vi "Set Pressure Units.vi"(8 "error in (no error)":errorcluster, 10 "Pressure Units (28: Pound-force pre square inch)":u32(ring)=28 items=["Unitless", "Frequency in units of hertz", "Frequency in units of kilohertz", "Frequency in units of megahertz", "Volts in units of microvolts", "Volts in units of millivolts", "Volts in units of volts", "Volts in units of kilovolts", "Current in units of microamperes", "Current in units of milliamps", "Current in units of amps", "Percent", "Parts-per-million", "Volts in units of decibels referenced to 1 milliwatt into 600 W load", "Resistance in units of ohms", "Resistance in units of kilohms", "Resistance in units of megohms", "Capacitance in units of nanofarads", "Capacitance in units of picofarads", "Capacitance in units of  microfarads", "Capacitance in units of millifarads", "Capacitance in units of farads", "Temperature in degrees Celsius", "Temperature in degrees Fahrenheit", "Period in units of nanoseconds", "Period in units of microseconds", "Period in units of milliseconds", "Period in units of seconds", "Pound-force pre square inch", "Meters of mercury", "Inches of mercury", "Inches of water", "Feet of water", "Meters of water", "Bar", "Pascal", "Grams per centimeter squared", "Inches of water @ 60 degrees Farhenheit", "Decibels"], 11 "VISA resource name":refnum<visa-resource-name>) -> (0 "error out":errorcluster, 3 "VISA resource name out":refnum<visa-resource-name>)   [LabVIEW 2011, in "Fluke 5XXX Series Multicalibrators.lvlib"]
doc: "This VI sets the pressure display units.\n\nNote:\n\nThis VI is available only for instrument model 5520A with option 700P (pressure modules)."
uses:
  Fluke 5XXX Series Multicalibrators.lvlib
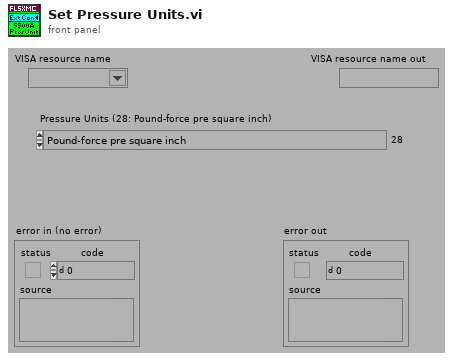
[diagram p1: front panel]
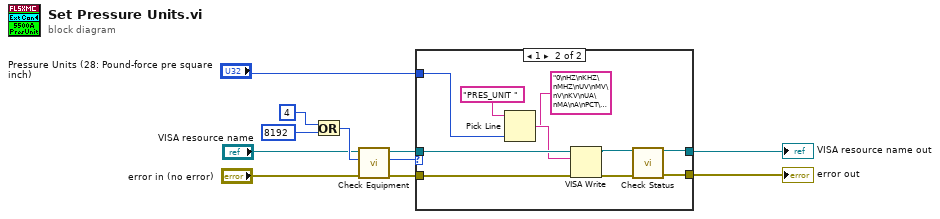
[diagram p0: block diagram]
diagram:
  n1 = Or(x=4 ("Numeric"), y=8192 ("Numeric")) -> (x .or. y?=w11:i32)
  n2 = call "Check Equipment.vi"("error in (no error)"="error in (no error)", "Bit Mask"=w11, "VISA resource name"="VISA resource name") -> ("error out"=w10:errorcluster, "Present?"=w9:u32, "VISA resource name out"=w8:refnum<visa-resource-name>)  [unwired: 6 in]
  n3 = case shown="1" w9 {
    tunnel: "Pressure Units (28: Pound-force pre square inch)" -> [_ w19]
    tunnel: [w12 w15] -> w4
    tunnel: w10 -> [w13 w22]
    tunnel: w8 -> [w12 w21]
    tunnel: [w13 w18] -> w5
    frame 0, Default {
    }
    frame 1 {
      n4 = Pick Line(string ("")="PRES_UNIT " ("Reset Command"), multi-line string="0\nHZ\nKHZ\nMHZ\nUV\nMV\nV\nKV\nUA\nMA\nA\nPCT\nPPM\nDBM\nOHM\nKOHM\nMOHM\nNF\nPF\nUF\nMF\nF\nCEL\nFAR\nNS\nUS\nMS\nS\nPSI\nMHG\nINHG\nINH2O\nFTH2O\nMH2O\nBAR\nPAL\nG/CM2\nINH2O60F\nDB", line index=w19) -> (output string=w20:string)
      n5 = VISA Write(VISA resource name=w21, write buffer=w20, error in (no error)=w22) -> (VISA resource name out=w16:refnum<visa-resource-name>, error out=w17:errorcluster)  [unwired: 1 out]
      n6 = call "Check Status.vi"("VISA resource name"=w16, "error in (no error)"=w17) -> ("VISA resource name out"=w15:refnum<visa-resource-name>, "error out"=w18:errorcluster)  [unwired: 12 in]
    }
  }
  "VISA resource name out" <- w4
  "error out" <- w5
